vi "Read Props.vi"(8 "error in (no error)":errorcluster, 11 "ImageButtonEditorPanel in":refnum<class "ImageButtonEditorPanel.lvclass">) -> (0 "error out":errorcluster, 2 "Props":T1, 3 "ImageButtonEditorPanel out":refnum<class "ImageButtonEditorPanel.lvclass">)   [LabVIEW 2020, in "VolatusGUIControls.lvlib" / "ImageButtonEditorPanel.lvclass"]
uses:
  ImageButtonEditorPanel.lvclass
  ImageButtonEditorPanel.lvclass/ImageButtonEditorPanel.ctl
  VolatusGUIControls.lvlib
  364b9c2f-6e96-453f-be81-99ceadfefcd6.vi
  JSON Props.ctl
  VolatusGUIEditorCore/Label Props.ctl
  VolatusGUIEditorCore/VolatusGUIEditorCore.lvlib
  VolatusGUIEditorCore/Position Props.ctl
  Props.ctl
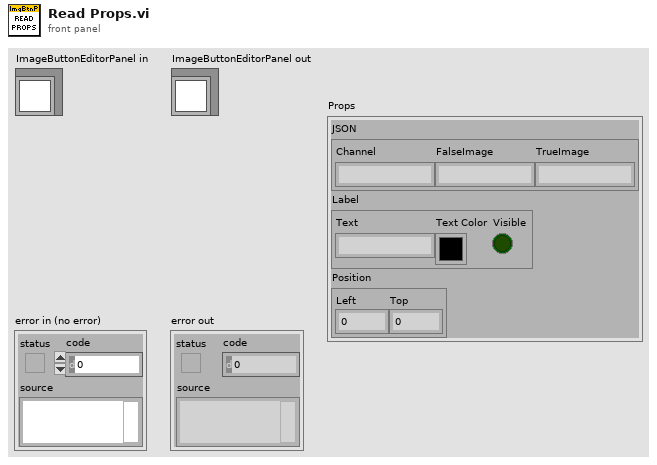
[diagram p1: front panel]
types:
  T1 = typedef "VolatusGUIControls.lvlib/ImageButtonEditorPanel.lvclass/Props.ctl" = cluster{"JSON":T2, "Label":T3, "Position":T4}
  T2 = typedef "VolatusGUIControls.lvlib/ImageButtonEditorPanel.lvclass/JSON Props.ctl" = cluster{"Channel":string, "FalseImage":string, "TrueImage":string}
  T3 = typedef "VolatusGUIEditorCore.lvlib/Label Props.ctl" = cluster{"Text":string, "Text Color":u32, "Visible":bool}
  T4 = typedef "VolatusGUIEditorCore.lvlib/Position Props.ctl" = cluster{"Left":i32, "Top":i32}
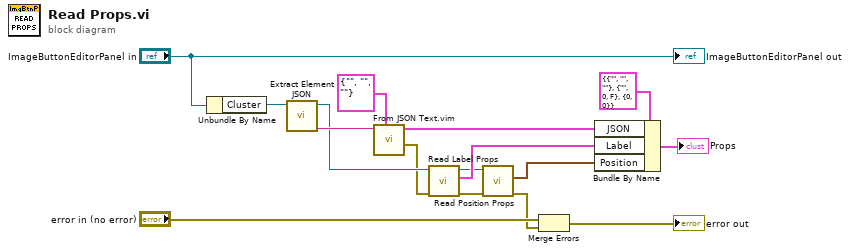
[diagram p0: block diagram]
diagram:
  n1 = Unbundle By Name("ImageButtonEditorPanel in") -> ("Cluster"=w14:refnum<vi>)
  n2 = call "Extract Element JSON.vi"("Ctl Refnum in"=w14) -> ("JSON"=w13:string, "Ctl Refnum"=w8:refnum<vi>)  [unwired: 7 in, 2 out]
  n3 = call "From JSON Text.vim"("Data Type and Default Value"=T2 {"Channel"="", "FalseImage"="", "TrueImage"=""} ("JSON Props"), "JSON"=w13) -> ("error out"=w7:errorcluster, "Data out"=w9:T2)  [unwired: 8 in]
  n4 = call "Read Label Props.vi"("error in (no error)"=w7, "Ctl Refnum in"=w8) -> ("error out"=w5:errorcluster, "Label Props"=w6:T3, "Ctl Refnum"=w4:refnum<vi>)  [unwired: 7 in]
  n5 = call "Read Position Props.vi"("error in (no error)"=w5, "Ctl Refnum in"=w4) -> ("error out"=w1:errorcluster, "Position Props"=w3:T4)  [unwired: 7 in, 1 out]
  n6 = Merge Errors("error in (no error)", w1) -> (→"error out":errorcluster)
  n7 = Bundle By Name(cluster=T1 {"JSON"={"Channel"="", "FalseImage"="", "TrueImage"=""}, "Label"={"Text"="", "Text Color"=0, "Visible"=FALSE}, "Position"={"Left"=0, "Top"=0}} ("Props"), "JSON"=w9, "Label"=w6, "Position"=w3) -> (→"Props":T1)
  "ImageButtonEditorPanel out" <- "ImageButtonEditorPanel in"
